vi "SubPanel_RFBlock_Panel_Rev11_v3.vi"(2 "error input":errorcluster, 3 "RF Block Input Array":T1[](array[typedef])) -> (0 "error output":errorcluster, 1 "RF Block Output Array":T1[](array[typedef]))   [LabVIEW 2019]
uses:
  Controls/RFBlockControl.ctl
panel:
  out "RF Block Output Echo":T1[](array[typedef])
  in  "VISA resource name":refnum<visa-resource-name>
  in  "Apply Configuration":bool
  in  "Frequency (GHz)":dbl
  in  "Power (dBm)":dbl
  out "Frequency (GHz) Output":dbl
  out "Power (dBm) Output":dbl
  in  "Power On?":bool
  in  "EXIT SUBVI":bool
  # "Instructions\nSelect Resource Under Name\nPower it on\nProvide the Frequency and Power desired\nPress \"Apply\"\nSee the output on the Echo above. If there are multiple devices configured, there will be multiple elements in the array"
  # "Nothing to see behind here"
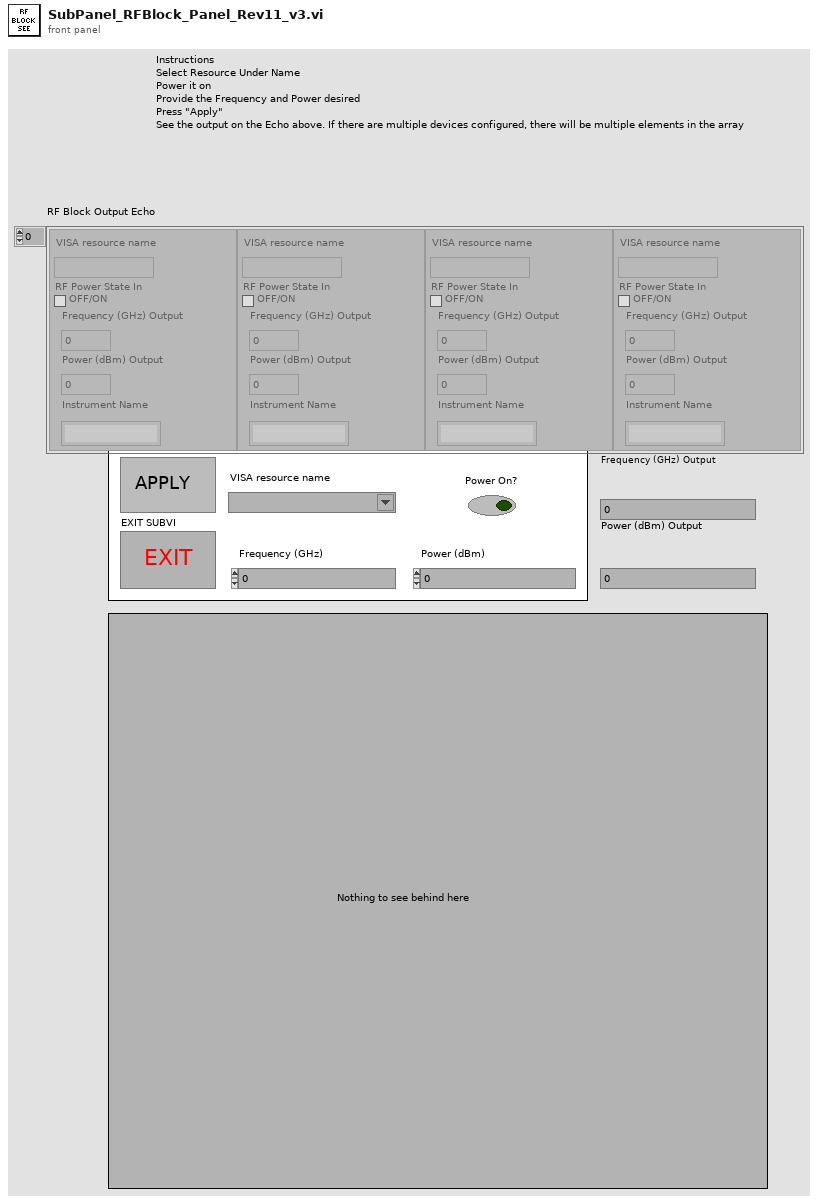
[diagram p1: front panel]
types:
  T1 = typedef "RFBlockControl.ctl" = cluster{"VISA resource name":refnum<visa-resource-name>, "RF Power State In":bool, "Frequency (GHz) Output":dbl, "Power (dBm) Output":dbl, "Instrument Name":string}
  T2 = cluster{"VISA resource name":refnum<visa-resource-name>, "Boolean out":bool, "Frequency (GHz) Output":dbl, "Power (dBm) Output":dbl, "Output Name":string}
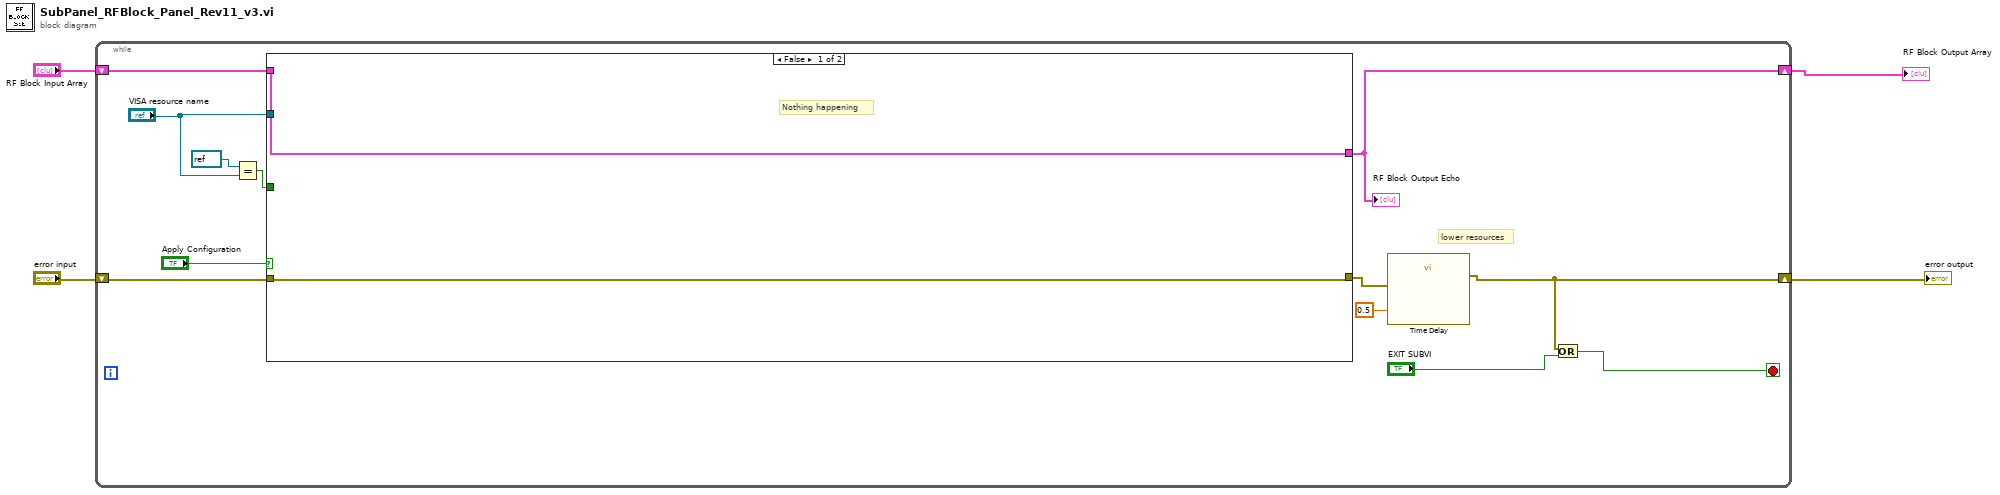
[diagram p0: block diagram]
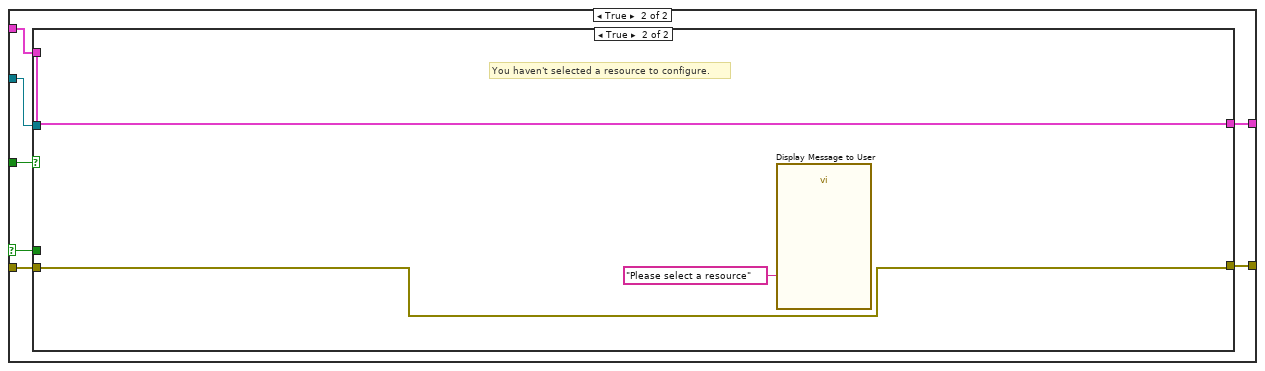
[diagram p2: hidden frame]
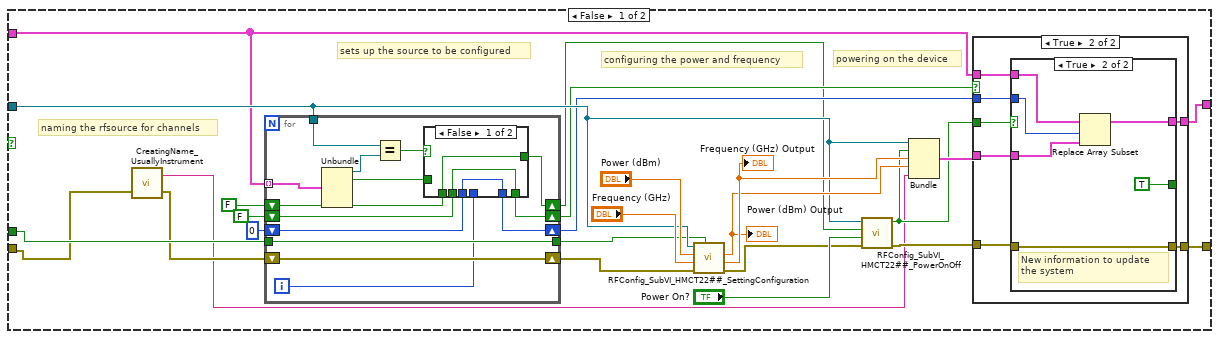
[diagram p3: hidden frame]
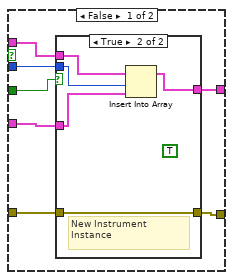
[diagram p4: hidden frame]
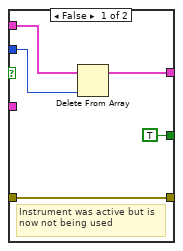
[diagram p6: hidden frame]
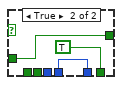
[diagram p7: hidden frame]
diagram:
  n1 = while {
    shift-right: [w7] -> w3
    shift-left: "error input" -> [w14]
    shift-right: [w8] -> w1
    shift-left: "RF Block Input Array" -> [w9]
    stop <- w5 stop-if-true
    # "lower resources"
    n2 = Equal?(x=refnum<visa-resource-name> refnum ("VISA resource name"), y="VISA resource name") -> (x = y?=w10:bool)
    n3 = case shown="False" "Apply Configuration" {
      selector: "Apply Configuration" -> [_ w22]
      tunnel: "VISA resource name" -> [_ w25]
      tunnel: [w18 w24] -> w13
      tunnel: w14 -> [w18 w23]
      tunnel: w10 -> [_ w21]
      tunnel: w9 -> [w17 w20]
      tunnel: [w17 w19] -> w8
      frame False {
        # "Nothing happening"
      }
      frame True {
        n4 = case shown="True" w21 {
          tunnel: w25 -> [w43 _]
          tunnel: [w35 w105] -> w24
          tunnel: w23 -> [w28 w105]
          tunnel: w22 -> [w32 _]
          tunnel: w20 -> [w40 w104]
          tunnel: [w33 w104] -> w19
          frame False {
            # "naming the rfsource for channels"
            # "powering on the device"
            # "configuring the power and frequency"
            # "sets up the source to be configured"
            n5 = call "CreatingName_UsuallyInstrument.vi"("error in (no error)"=w28) -> ("error in (no error) 2"=w27:errorcluster, "Output Name"=w26:string)  [unwired: 1 in]
            n6 = for {
              tunnel: w40 -> [w96] mode=indexing
              shift-right: [w90] -> w44
              shift-left: w27 -> [w90]
              tunnel: w43 -> [w94]
              shift-right: [w91] -> w38
              shift-left: FALSE -> [w92]
              shift-right: [w85] -> w37
              shift-left: 0 -> [w86]
              tunnel: w32 -> [w89]
              tunnel: [w89] -> w31
              shift-right: [w83] -> w29
              shift-left: FALSE -> [w87]
              i -> [w84]
              n7 = Unbundle(w96) -> ("VISA resource name"=w95:refnum<visa-resource-name>, "RF Power State In"=w88:bool)  [unwired: 3 out]
              n8 = Equal?(x=w94, y=w95) -> (x = y?=w93:bool)
              n9 = case shown="False" w93 {
                tunnel: w92 -> [w99 _]
                tunnel: [w99 TRUE] -> w91
                tunnel: w88 -> [_ w100]
                tunnel: w87 -> [w97 _]
                tunnel: w86 -> [w98 _]
                tunnel: [w98 w101] -> w85
                tunnel: w84 -> [_ w101]
                tunnel: [w97 w100] -> w83
                frame False {
                }
                frame True {
                }
              }
            }
            n10 = call "RFConfig_SubVI_HMCT22##_SettingConfiguration.vi"("Apply Configurations"=w31, "error in (no error)"=w44, "Frequency (GHz)"="Frequency (GHz)", "Power (dBm)"="Power (dBm)", "VISA Refnum in"=w43) -> ("error out"=w47:errorcluster, "Frequency (GHz) Output"=w46:dbl, "Power (dBm) Output"=w45:dbl)  [unwired: 4 in]
            "Frequency (GHz) Output" <- w46
            "Power (dBm) Output" <- w45
            n11 = call "RFConfig_SubVI_HMCT22##_PowerOnOff.vi"("error in (no error)"=w47, "Power On?"="Power On?", "Boolean in"=w29, "VISA Refnum in"=w43) -> ("error out"=w36:errorcluster, "Boolean out"=w34:bool)  [unwired: 6 in]
            n12 = Bundle("VISA resource name"=w43, "Boolean out"=w34, "Frequency (GHz) Output"=w46, "Power (dBm) Output"=w45, "Output Name"=w26) -> (w39:T2)  [unwired: 1 in]
            n13 = case shown="True" w38 {
              tunnel: w40 -> [w56 w67]
              tunnel: w39 -> [w55 w65]
              tunnel: w37 -> [w54 w68]
              tunnel: w36 -> [w51 w70]
              tunnel: [w52 w71] -> w35
              tunnel: w34 -> [w57 w69]
              tunnel: [w53 w66] -> w33
              frame False {
                n14 = case shown="True" w57 {
                  tunnel: w56 -> [w58 w64]
                  tunnel: w55 -> [_ w63]
                  tunnel: w54 -> [_ w62]
                  tunnel: [w58 w61] -> w53
                  tunnel: [w59 w60] -> w52
                  tunnel: w51 -> [w59 w60]
                  frame False {
                    # "No instrument initialized and not powered on. Instrument not active"
                  }
                  frame True {
                    (unwired) TRUE
                    # "New Instrument Instance"
                    n15 = Insert Into Array(array=w64, index=w62, new element=w63) -> (w61:T1[])
                  }
                }
              }
              frame True {
                n16 = case shown="True" w69 {
                  tunnel: [w76 w82] -> w71
                  tunnel: w70 -> [w76 w82]
                  tunnel: w68 -> [w75 w80]
                  tunnel: w67 -> [w74 w81]
                  tunnel: [w73 w78] -> w66
                  tunnel: w65 -> [_ w79]
                  tunnel: [TRUE TRUE] -> _
                  frame False {
                    # "Instrument was active but is now not being used"
                    n17 = Delete From Array(array=w74, index=w75) -> (array with subset deleted=w73:T1[])  [unwired: 1 in, 1 out]
                  }
                  frame True {
                    # "New information to update the system"
                    n18 = Replace Array Subset(array=w81, new element=w79, index=w80) -> (w78:T1[])
                  }
                }
              }
            }
          }
          frame True {
            # "You haven't selected a resource to configure."
            n19 = call "Display Message to User"("Message"="Please select a resource") -> ()  [unwired: 9 in, 2 out]
          }
        }
      }
    }
    "RF Block Output Echo" <- w8
    n20 = call "Time Delay"("error in (no error)"=w13, "Delay Time (s)"=0.5) -> ("error out"=w7:errorcluster)  [unwired: 9 in]
    n21 = Or(x=w7, y="EXIT SUBVI") -> (x .or. y?=w5:bool)
  }
  "error output" <- w3
  "RF Block Output Array" <- w1
